vi "ConvertToCartesianVector.vi"(8 "error in (no error)":errorcluster, 11 "PolarVector in":refnum<class "PolarVector.lvclass">) -> (0 "error out":errorcluster, 3 "CartesianVector.lvclass":refnum<class "CartesianVector.lvclass">)   [LabVIEW 2011, in "PolarVector.lvclass"]
doc: "Converts polar vectors to cartesian vectors."
uses:
  PolarVector.lvclass
  CartesianVector/CartesianVector.lvclass
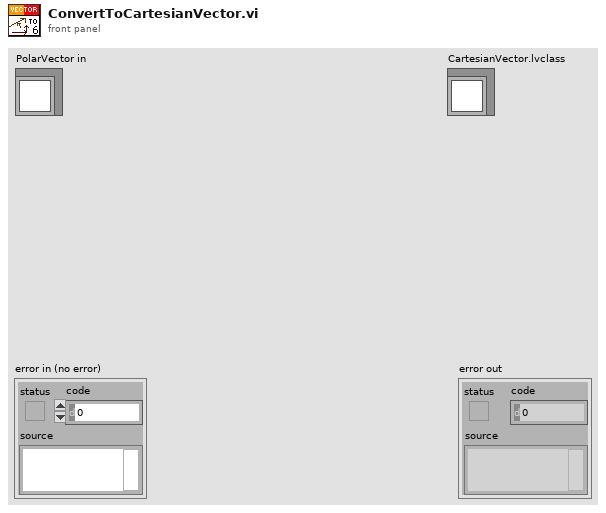
[diagram p1: front panel]
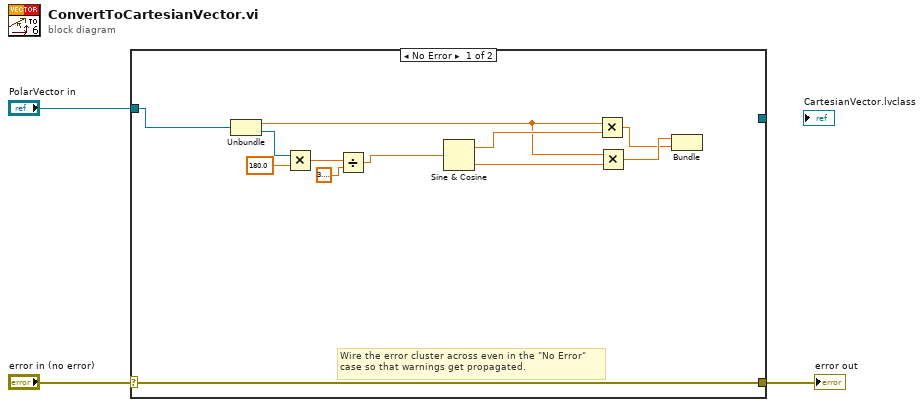
[diagram p0: block diagram]
diagram:
  n1 = case shown="No Error" "error in (no error)" {
    selector: "error in (no error)" -> [w15 w17]
    tunnel: [w15 w17] -> w2
    tunnel: "PolarVector in" -> [w14 w16]
    tunnel: [_ w16] -> _
    frame No Error {
      # "Wire the error cluster across even in the \"No Error\"\ncase so that warnings get propagated."
      n2 = Unbundle(w14) -> (w12:dbl, w5:refnum<class "Angle.lvclass">)
      n3 = Multiply(x=w5, y=180.0) -> (x*y=w7:dbl)
      n4 = Divide(x=w7, y=3.141592653589793) -> (x/y=w6:dbl)
      n5 = Sine & Cosine(0:w6) -> (1:w13:dbl, 2:w11:dbl)
      n6 = Multiply(x=w12, y=w13) -> (x*y=w9:dbl)
      n7 = Multiply(x=w12, y=w11) -> (x*y=w10:dbl)
      n8 = Bundle(w10, w9) -> ()  [unwired: 1 in, 1 out]
    }
    frame Error {
    }
  }
  "error out" <- w2
